vi "PumpValve2.vi"() -> ()   [LabVIEW 2015]
uses:
  PumpValve.ctl
  <vilib>/DAQmx/write.llb/DAQmx Write (Digital 1D Bool NChan 1Samp 1Line).vi
  <vilib>/DAQmx/miscellaneous.llb/DAQmx Fill In Error Info.vi
panel:
  out "Tank":dbl(slide) scale=0.0..100.0
  in  "Drain Time(ms)":dbl
  in  "Fill Time(ms)":dbl
  in  "stop":bool
  in  "Pause Button":bool
  in  "Drain":bool
  in  "Stop Program":bool
  in  "Fill":bool
  out "Current State":T1
  in  "Pump 2":bool
  in  "Blue Valve":bool
  in  "Green Valve":bool
  out "Green":i32
  out "Blue":i32
  out "Pump":i32
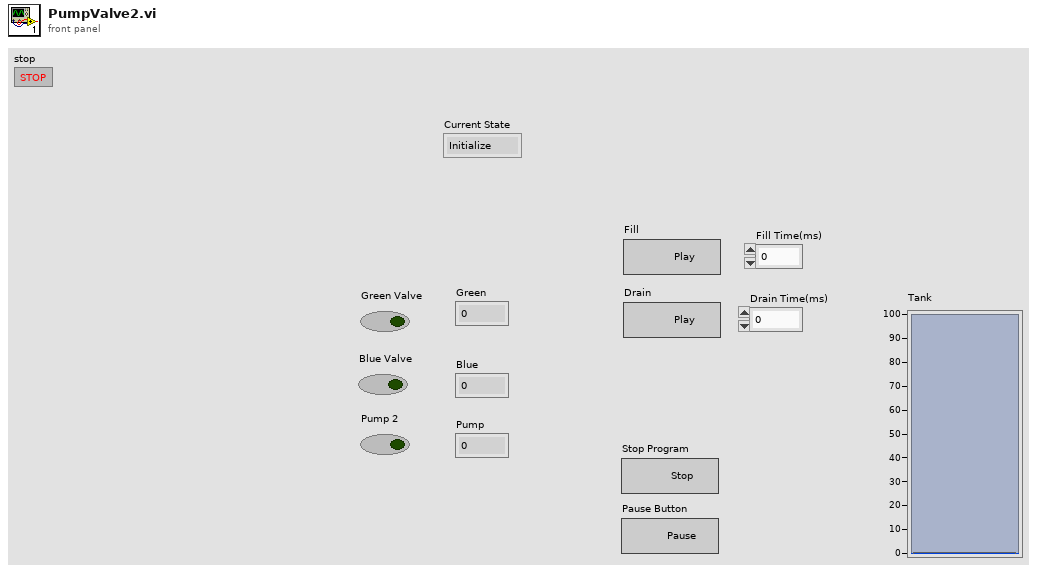
[diagram p1: front panel]
types:
  T1 = typedef "PumpValve.ctl" = enum16{"Initialize", "Idle", "Fill", "Drain", "Stop"}
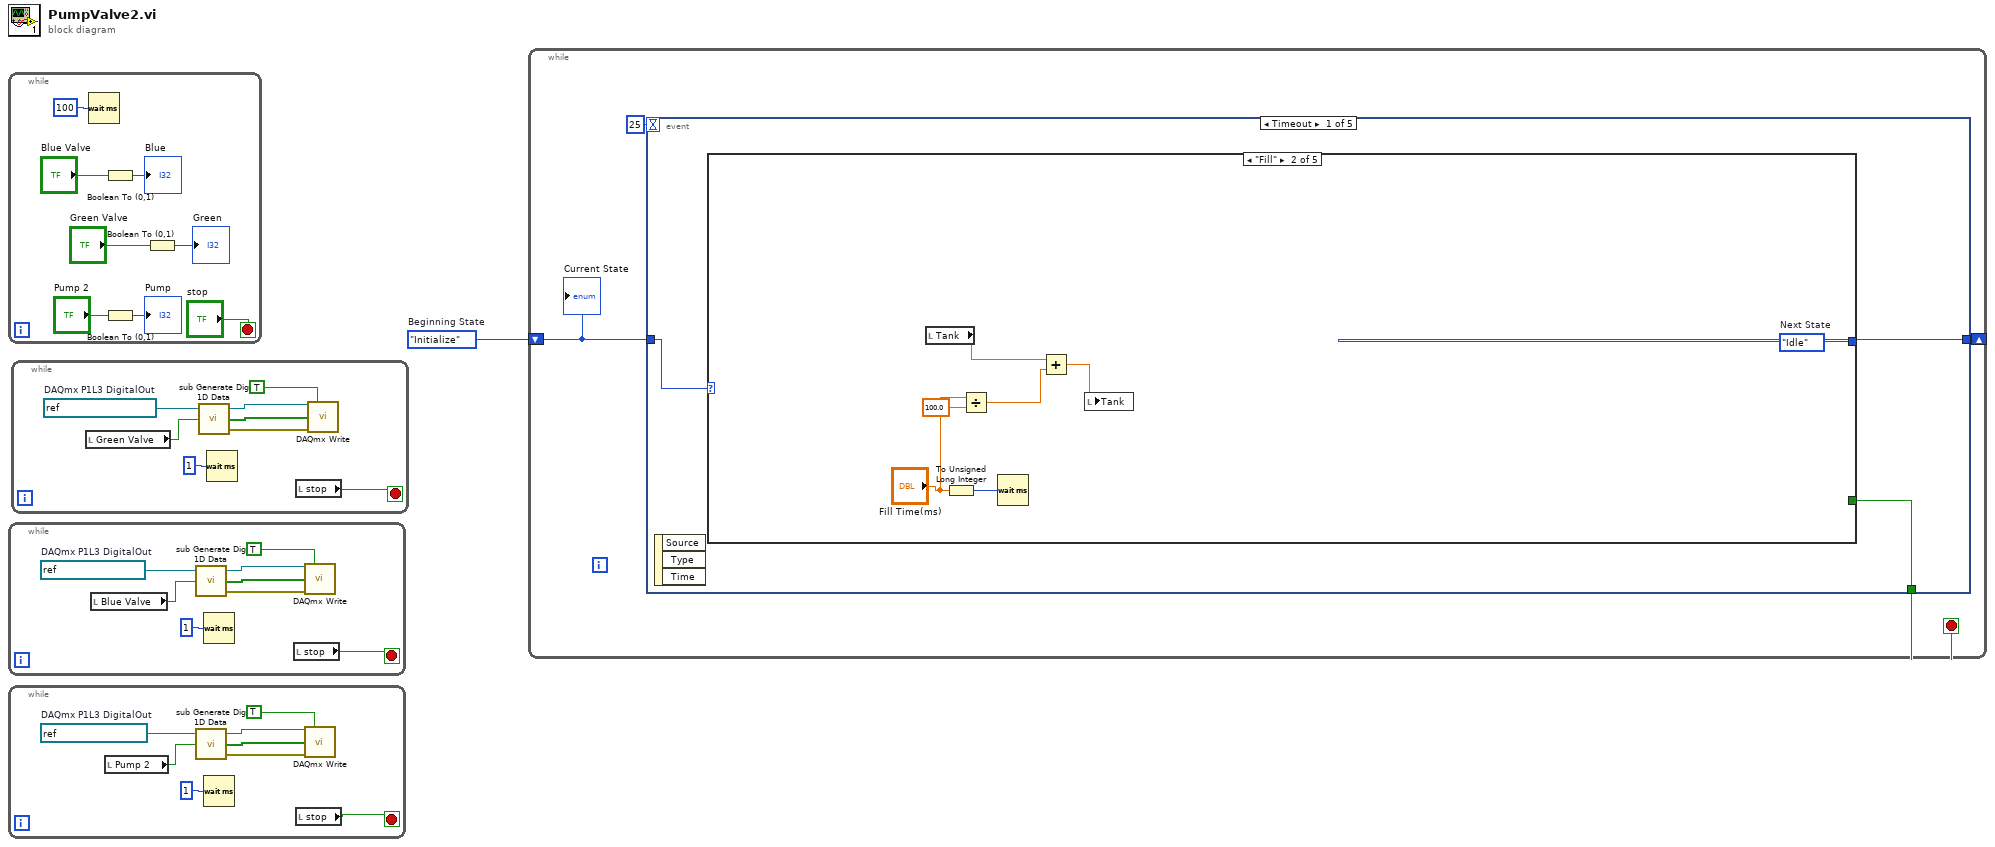
[diagram p0: block diagram]
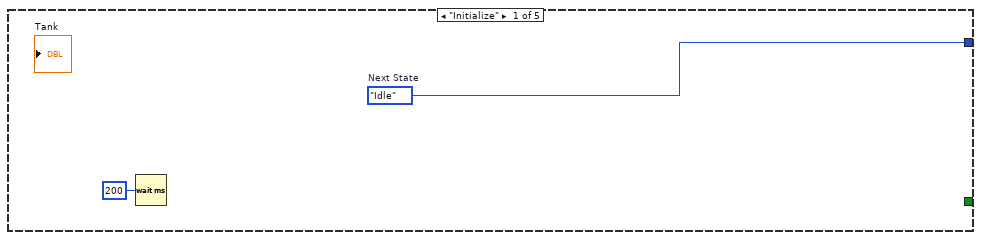
[diagram p2: hidden frame]
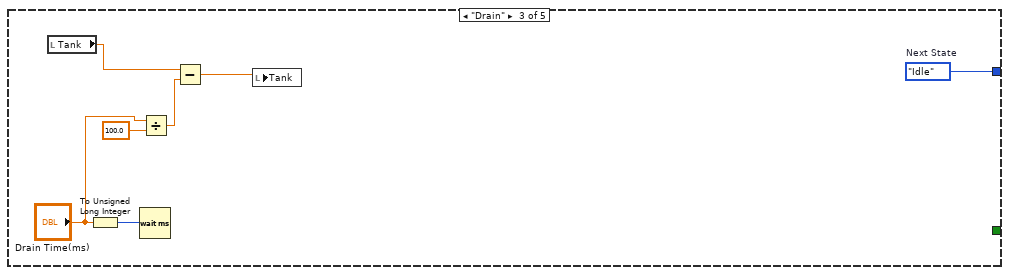
[diagram p3: hidden frame]
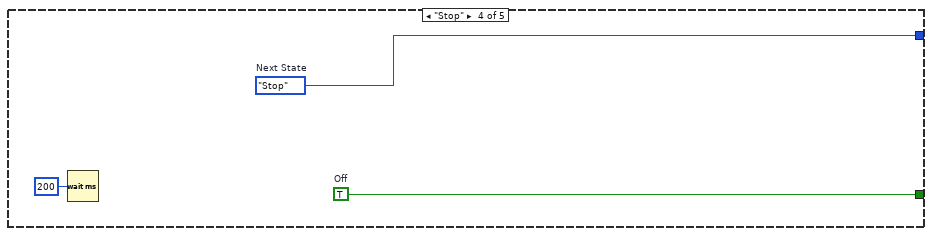
[diagram p4: hidden frame]
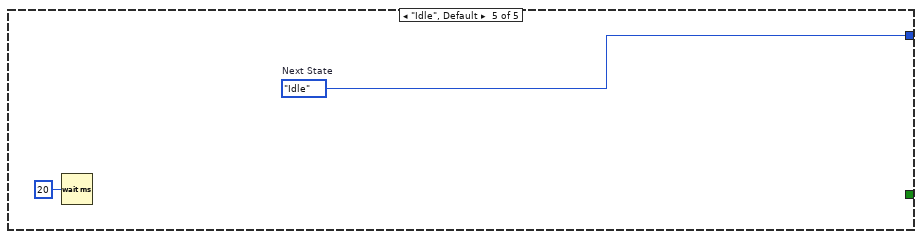
[diagram p5: hidden frame]
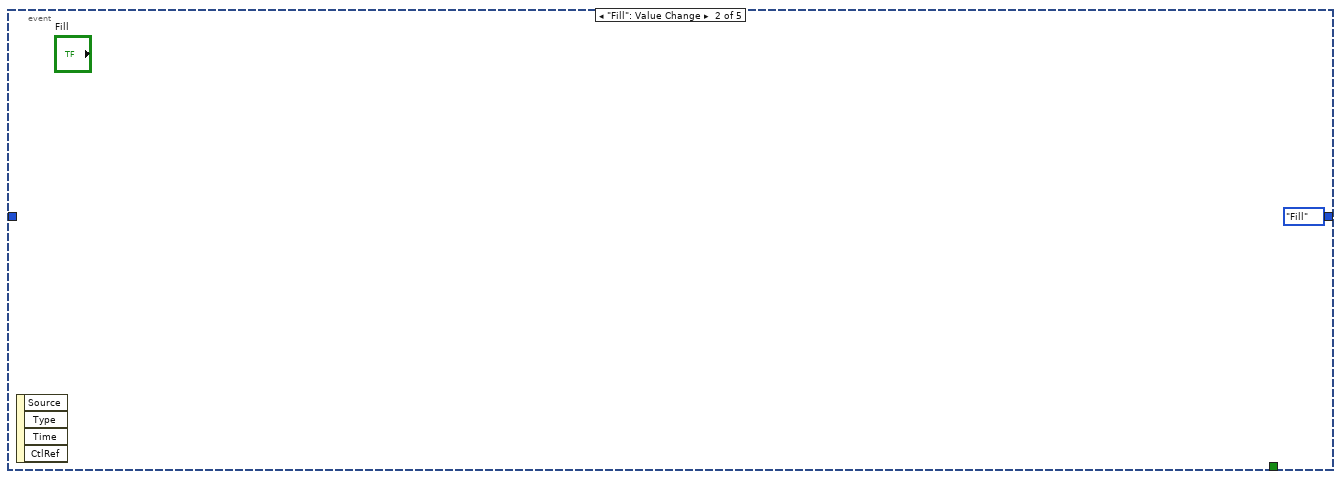
[diagram p6: hidden frame]
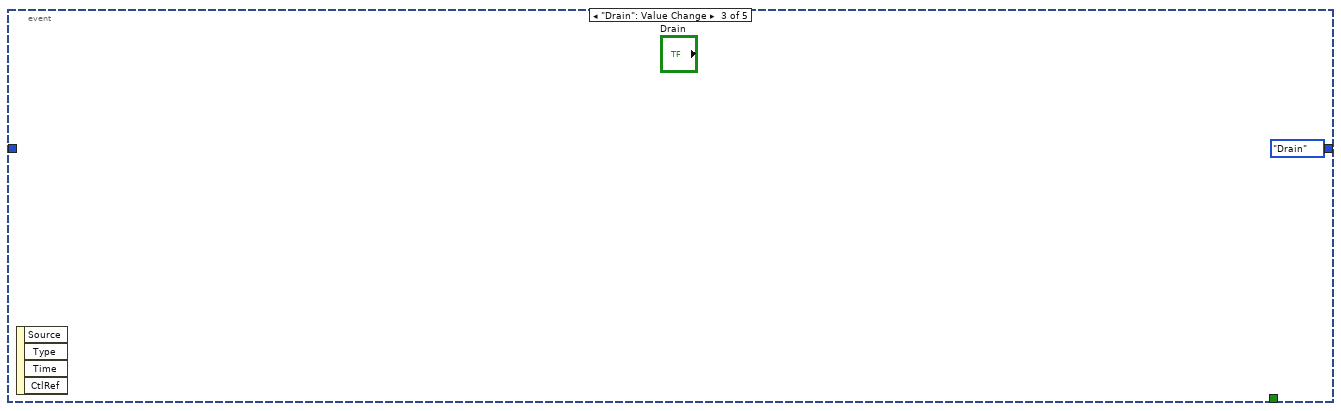
[diagram p7: hidden frame]
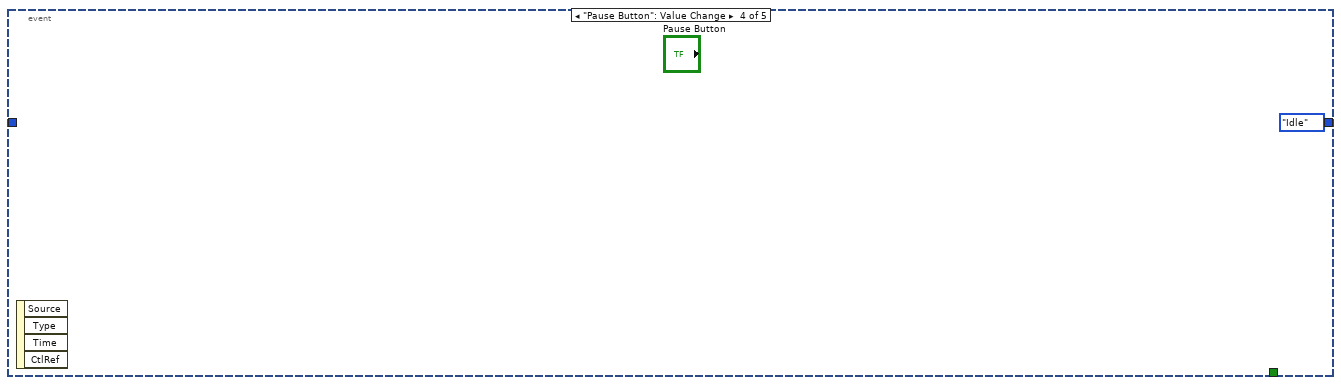
[diagram p8: hidden frame]
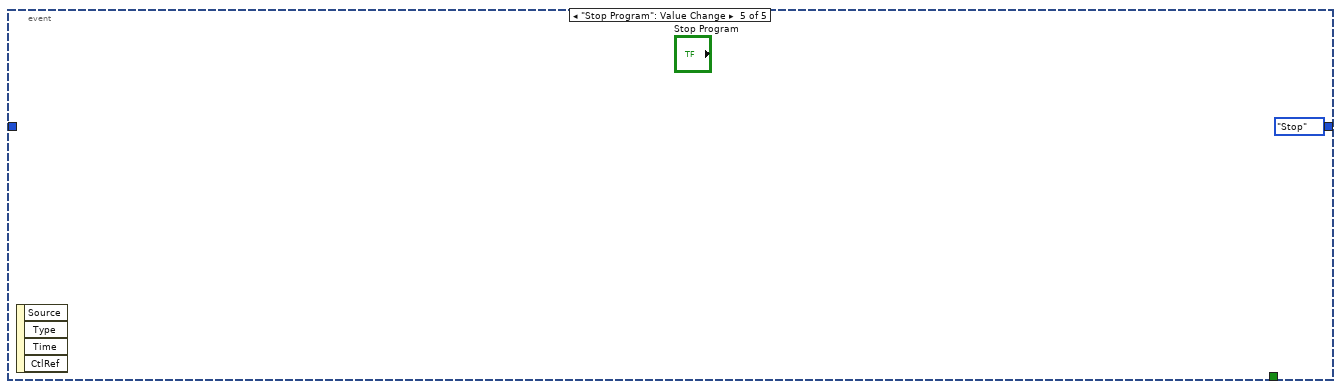
[diagram p9: hidden frame]
diagram:
  w1 = PumpValve."Initialize"  # Beginning State
  n1 = while {
    stop <- "stop" stop-if-true
    n2 = Wait (ms)(milliseconds to wait=u32 100) -> ()  [unwired: 1 out]
    n3 = Boolean To (0,1)(Boolean="Blue Valve") -> (0, 1=→"Blue":i16)
    n4 = Boolean To (0,1)(Boolean="Pump 2") -> (0, 1=→"Pump":i16)
    n5 = Boolean To (0,1)(Boolean="Green Valve") -> (0, 1=→"Green":i16)
  }
  n6 = while {
    stop <- w10 stop-if-true
    w17 = refnum<k21> "DigitalOutBlue"  # DAQmx P1L3 DigitalOut
    n7 = local read "Blue Valve"() -> (w11:bool)
    n8 = call <vilib>:"sub Generate Dig 1D Data.vi"("initial value"=w11, "task in"=w17) -> ("error out"=w14:errorcluster, "Data"=w15:bool[], "task out"=w16:refnum<k21>)  [unwired: 1 in]
    n9 = Wait (ms)(milliseconds to wait=u32 1) -> ()  [unwired: 1 out]
    n10 = local read "stop"() -> (w10:bool)
    n11 = call-poly <vilib>:"DAQmx Write.vi"("task/channels in"=w16, "auto start"=TRUE, "data"=w15, "error in"=w14) -> ()  [unwired: 9 in, 3 out]
  }
  n12 = while {
    stop <- w18 stop-if-true
    w25 = refnum<k21> "P0L0DigitalOut"  # DAQmx P1L3 DigitalOut
    n13 = local read "Pump 2"() -> (w19:bool)
    n14 = call <vilib>:"sub Generate Dig 1D Data.vi"("initial value"=w19, "task in"=w25) -> ("error out"=w22:errorcluster, "Data"=w23:bool[], "task out"=w24:refnum<k21>)  [unwired: 1 in]
    n15 = Wait (ms)(milliseconds to wait=u32 1) -> ()  [unwired: 1 out]
    n16 = local read "stop"() -> (w18:bool)
    n17 = call-poly <vilib>:"DAQmx Write.vi"("task/channels in"=w24, "auto start"=TRUE, "data"=w23, "error in"=w22) -> ()  [unwired: 9 in, 3 out]
  }
  n18 = while {
    stop <- w26 stop-if-true
    w33 = refnum<k21> "DigitalOutGreen"  # DAQmx P1L3 DigitalOut
    n19 = local read "Green Valve"() -> (w27:bool)
    n20 = call <vilib>:"sub Generate Dig 1D Data.vi"("initial value"=w27, "task in"=w33) -> ("error out"=w30:errorcluster, "Data"=w31:bool[], "task out"=w32:refnum<k21>)  [unwired: 1 in]
    n21 = Wait (ms)(milliseconds to wait=u32 1) -> ()  [unwired: 1 out]
    n22 = local read "stop"() -> (w26:bool)
    n23 = call-poly <vilib>:"DAQmx Write.vi"("task/channels in"=w32, "auto start"=TRUE, "data"=w31, "error in"=w30) -> ()  [unwired: 9 in, 3 out]
  }
  n24 = while {
    shift-right: [w35] -> _
    shift-left: w1 -> [w37]
    stop <- w34 stop-if-true
    n25 = event shown="[0] Timeout" {
      selector: _ -> [_ _ _ _ _]
      dyn-events: _ -> [_ _ _ _ _]
      timeout: 25 -> [_ _ _ _ _]
      tunnel: w37 -> [w40 _ _ _ _]
      tunnel: [w39 PumpValve."Fill" ("Next State") PumpValve."Drain" ("Next State") PumpValve."Idle" ("Next State") PumpValve."Stop" ("Next State")] -> w35
      tunnel: [w38 _ _ _ _] -> w34
      event Timeout {
        n26 = event-data() -> ()  [unwired: 1 in, 3 out]
        n27 = case shown="\"Fill\"" w40 {
          tunnel: [w42 w49 w56 w59 w61] -> w39
          tunnel: [_ _ _ w57 _] -> w38
          frame "Initialize" {
            w42 = PumpValve."Idle"  # Next State
            n28 = Wait (ms)(milliseconds to wait=u32 200) -> ()  [unwired: 1 out]
          }
          frame "Fill" {
            w49 = PumpValve."Idle"  # Next State
            n29 = local read "Tank"() -> (w44:dbl)
            n30 = To Unsigned Long Integer(number="Fill Time(ms)") -> (unsigned 32bit integer=w48:u32)
            n31 = Divide(x="Fill Time(ms)", y=100.0) -> (x/y=w45:dbl)
            n32 = Wait (ms)(milliseconds to wait=w48) -> ()  [unwired: 1 out]
            n33 = Add(x=w44, y=w45) -> (x+y=w43:dbl)
            n34 = local write "Tank"(w43) -> ()
          }
          frame "Drain" {
            w56 = PumpValve."Idle"  # Next State
            n35 = local read "Tank"() -> (w52:dbl)
            n36 = To Unsigned Long Integer(number="Drain Time(ms)") -> (unsigned 32bit integer=w55:u32)
            n37 = Wait (ms)(milliseconds to wait=w55) -> ()  [unwired: 1 out]
            n38 = Divide(x="Drain Time(ms)", y=100.0) -> (x/y=w51:dbl)
            n39 = Subtract(x=w52, y=w51) -> (x-y=w50:dbl)
            n40 = local write "Tank"(w50) -> ()
          }
          frame "Stop" {
            w57 = TRUE  # Off
            w59 = PumpValve."Stop"  # Next State
            n41 = Wait (ms)(milliseconds to wait=u32 200) -> ()  [unwired: 1 out]
          }
          frame "Idle", Default {
            w61 = PumpValve."Idle"  # Next State
            n42 = Wait (ms)(milliseconds to wait=u32 20) -> ()  [unwired: 1 out]
          }
        }
      }
      event "Fill": Value Change {
        n43 = event-data() -> ()  [unwired: 1 in, 4 out]
      }
      event "Drain": Value Change {
        n44 = event-data() -> ()  [unwired: 1 in, 4 out]
      }
      event "Pause Button": Value Change {
        n45 = event-data() -> ()  [unwired: 1 in, 4 out]
      }
      event "Stop Program": Value Change {
        n46 = event-data() -> ()  [unwired: 1 in, 4 out]
      }
    }
    "Current State" <- w37
  }
